vi "PowerLineChannel.vi"(0 "Power Line\nConfigurations":T1[](array[typedef]) {"Max Current [A]" format="%#_13g"; "Min Current [A]" format="%#_13g"; "Shunt Resistor [Ohm]" format="%#_13g"}, 2 "ADC Available":i32=8, 3 "ADC Sampling Rates":dbl[](array[numeric])=[2000000.0, 2000000.0, 200000.0, 133000.0, 100000.0, 2000000.0, 2000000.0, 200000.0, 133000.0, 100000.0]) -> (7 "Output Task":refnum<k21>, 8 "Sampling Rate":dbl, 10 "Output Error":errorcluster)   [LabVIEW 2020]
uses:
  HiFiveUnmatchedPowerLineConfig.ctl
  305589ae-c1bd-4c9d-bca7-de63f4121e79.vi
  <vilib>/DAQmx/create/channels.llb/DAQmx Create Channel (AI-Current-Basic).vi
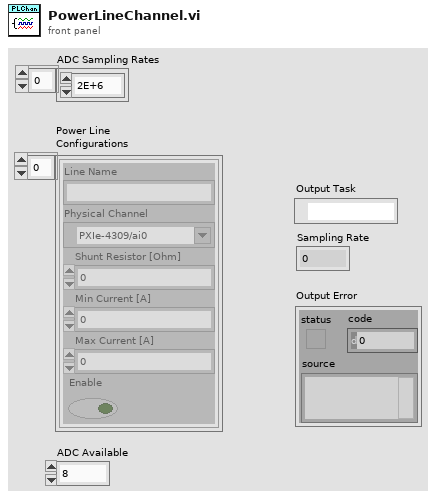
[diagram p1: front panel]
types:
  T1 = typedef "HiFiveUnmatchedPowerLineConfig.ctl" = cluster{"Line Name":string, "Physical Channel":tag, "Shunt Resistor [Ohm]":dbl, "Min Current [A]":dbl, "Max Current [A]":dbl, "Enable":bool}
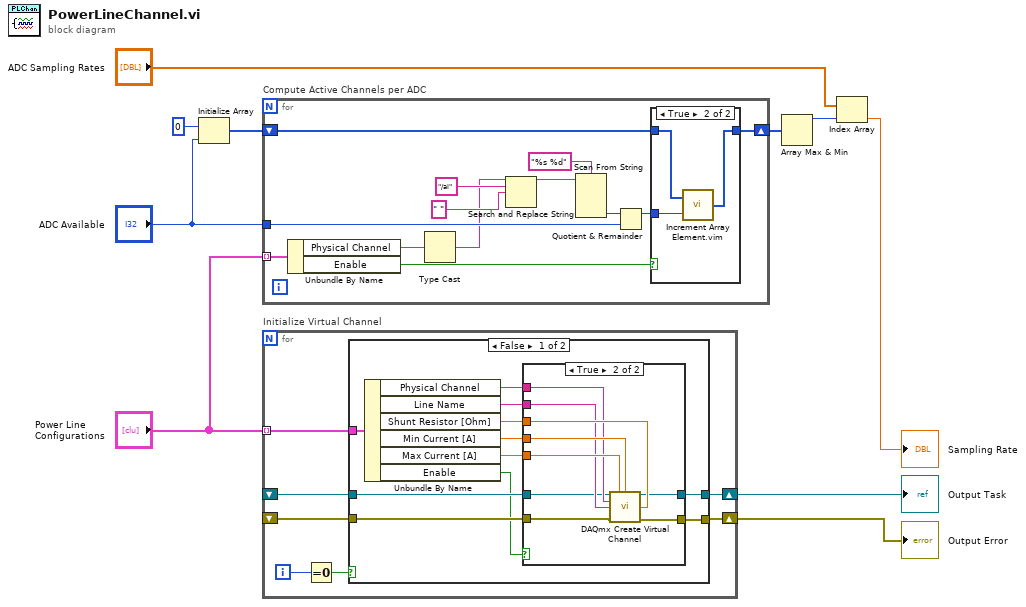
[diagram p0: block diagram]
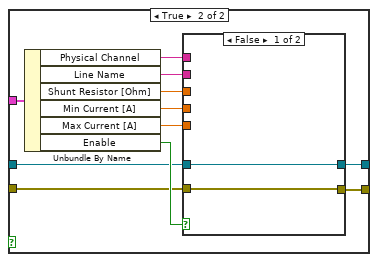
[diagram p4: hidden frame]
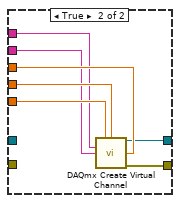
[diagram p5: hidden frame]
diagram:
  n1 = Initialize Array(0 ("element"), "ADC Available") -> (w8:i32[])
  n2 = for "Compute Active Channels per ADC" {
    tunnel: "Power Line\nConfigurations" -> [w23] mode=indexing
    shift-right: [w19] -> w7
    shift-left: w8 -> [w20]
    tunnel: "ADC Available" -> [w17]
    n3 = Unbundle By Name(w23) -> ("Physical Channel"=w22:tag, "Enable"=w21:bool)
    n4 = Type Cast(x=w22) -> (*(type *) &x=w12:string)  [unwired: 1 in]
    n5 = Search and Replace String(input string=w12, search string="/ai", replace string=" " ("replace string (\"\")")) -> (result string=w11:string)  [unwired: 5 in, 3 out]
    n6 = Scan From String(format string="%s %d", input string=w11) -> (output 2=w15:i32)  [unwired: 5 in, 3 out]
    n7 = Quotient & Remainder(x=w15, y=w17) -> (x-y*floor(x/y)=w16:i32)  [unwired: 1 out]
    n8 = case shown="True" w21 {
      tunnel: w20 -> [w24 w27]
      tunnel: [w24 w26] -> w19
      tunnel: w16 -> [_ w25]
      frame False {
      }
      frame True {
        n9 = call "Increment Array Element.vim"("index"=w25, "array in"=w27) -> ("array out"=w26:i32[])
      }
    }
  }
  n10 = for "Initialize Virtual Channel" {
    tunnel: "Power Line\nConfigurations" -> [w34] mode=indexing
    shift-right: [w33] -> w3
    shift-left: _ -> [w29]
    shift-right: [w32] -> w2
    shift-left: _ -> [w28]
    i -> [w30]
    n11 = Equal To 0?(x=w30) -> (x = 0?=w31:bool)
    n12 = case shown="False" w31 {
      tunnel: w34 -> [w38 w67]
      tunnel: [w40 w61] -> w33
      tunnel: [w39 w60] -> w32
      tunnel: w29 -> [w37 w58]
      tunnel: w28 -> [w36 w57]
      frame False {
        n13 = Unbundle By Name(w38) -> ("Physical Channel"=w41:tag, "Line Name"=w42:string, "Shunt Resistor [Ohm]"=w43:dbl, "Min Current [A]"=w44:dbl, "Max Current [A]"=w45:dbl, "Enable"=w35:bool)
        n14 = case shown="True" w35 {
          tunnel: w45 -> [_ w56]
          tunnel: w44 -> [_ w55]
          tunnel: w43 -> [_ w54]
          tunnel: w42 -> [_ w53]
          tunnel: w41 -> [_ w52]
          tunnel: [w47 w51] -> w40
          tunnel: [w46 w50] -> w39
          tunnel: w37 -> [w47 w49]
          tunnel: w36 -> [w46 w48]
          frame False {
          }
          frame True {
            n15 = call-poly <vilib>:"DAQmx Create Virtual Channel.vi"("task in"=w49, "maximum value"=w56, "minimum value"=w55, "physical channels"=w52, "name to assign"=w53, "external shunt resistor value"=w54, "error in"=w48) -> ("task out"=w51:refnum<k21>, "error out"=w50:errorcluster)  [unwired: 7 in]
          }
        }
      }
      frame True {
        n16 = Unbundle By Name(w67) -> ("Physical Channel"=w66:tag, "Line Name"=w65:string, "Shunt Resistor [Ohm]"=w64:dbl, "Min Current [A]"=w63:dbl, "Max Current [A]"=w62:dbl, "Enable"=w59:bool)
        n17 = case shown="False" w59 {
          tunnel: w62 -> [_ w76]
          tunnel: w63 -> [_ w75]
          tunnel: w64 -> [_ w74]
          tunnel: w65 -> [_ w73]
          tunnel: w66 -> [_ w72]
          tunnel: [w69 w71] -> w61
          tunnel: [w68 w70] -> w60
          tunnel: w58 -> [w69 _]
          tunnel: w57 -> [w68 _]
          frame False {
          }
          frame True {
            n18 = call-poly <vilib>:"DAQmx Create Virtual Channel.vi"("maximum value"=w76, "minimum value"=w75, "physical channels"=w72, "name to assign"=w73, "external shunt resistor value"=w74) -> ("task out"=w71:refnum<k21>, "error out"=w70:errorcluster)  [unwired: 9 in]
          }
        }
      }
    }
  }
  "Output Error" <- w2
  "Output Task" <- w3
  n19 = Array Max & Min(array=w7) -> (max value=w4:i32)  [unwired: 3 out]
  n20 = Index Array(array="ADC Sampling Rates", index=w4) -> (element=→"Sampling Rate":dbl)
